vi "CRYSet Recall Front Panel.vi"(11 "Vi Ref":refnum<vi>) -> ()   [LabVIEW 2013]
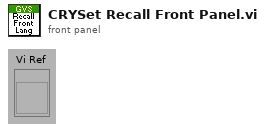
[diagram p1: front panel]
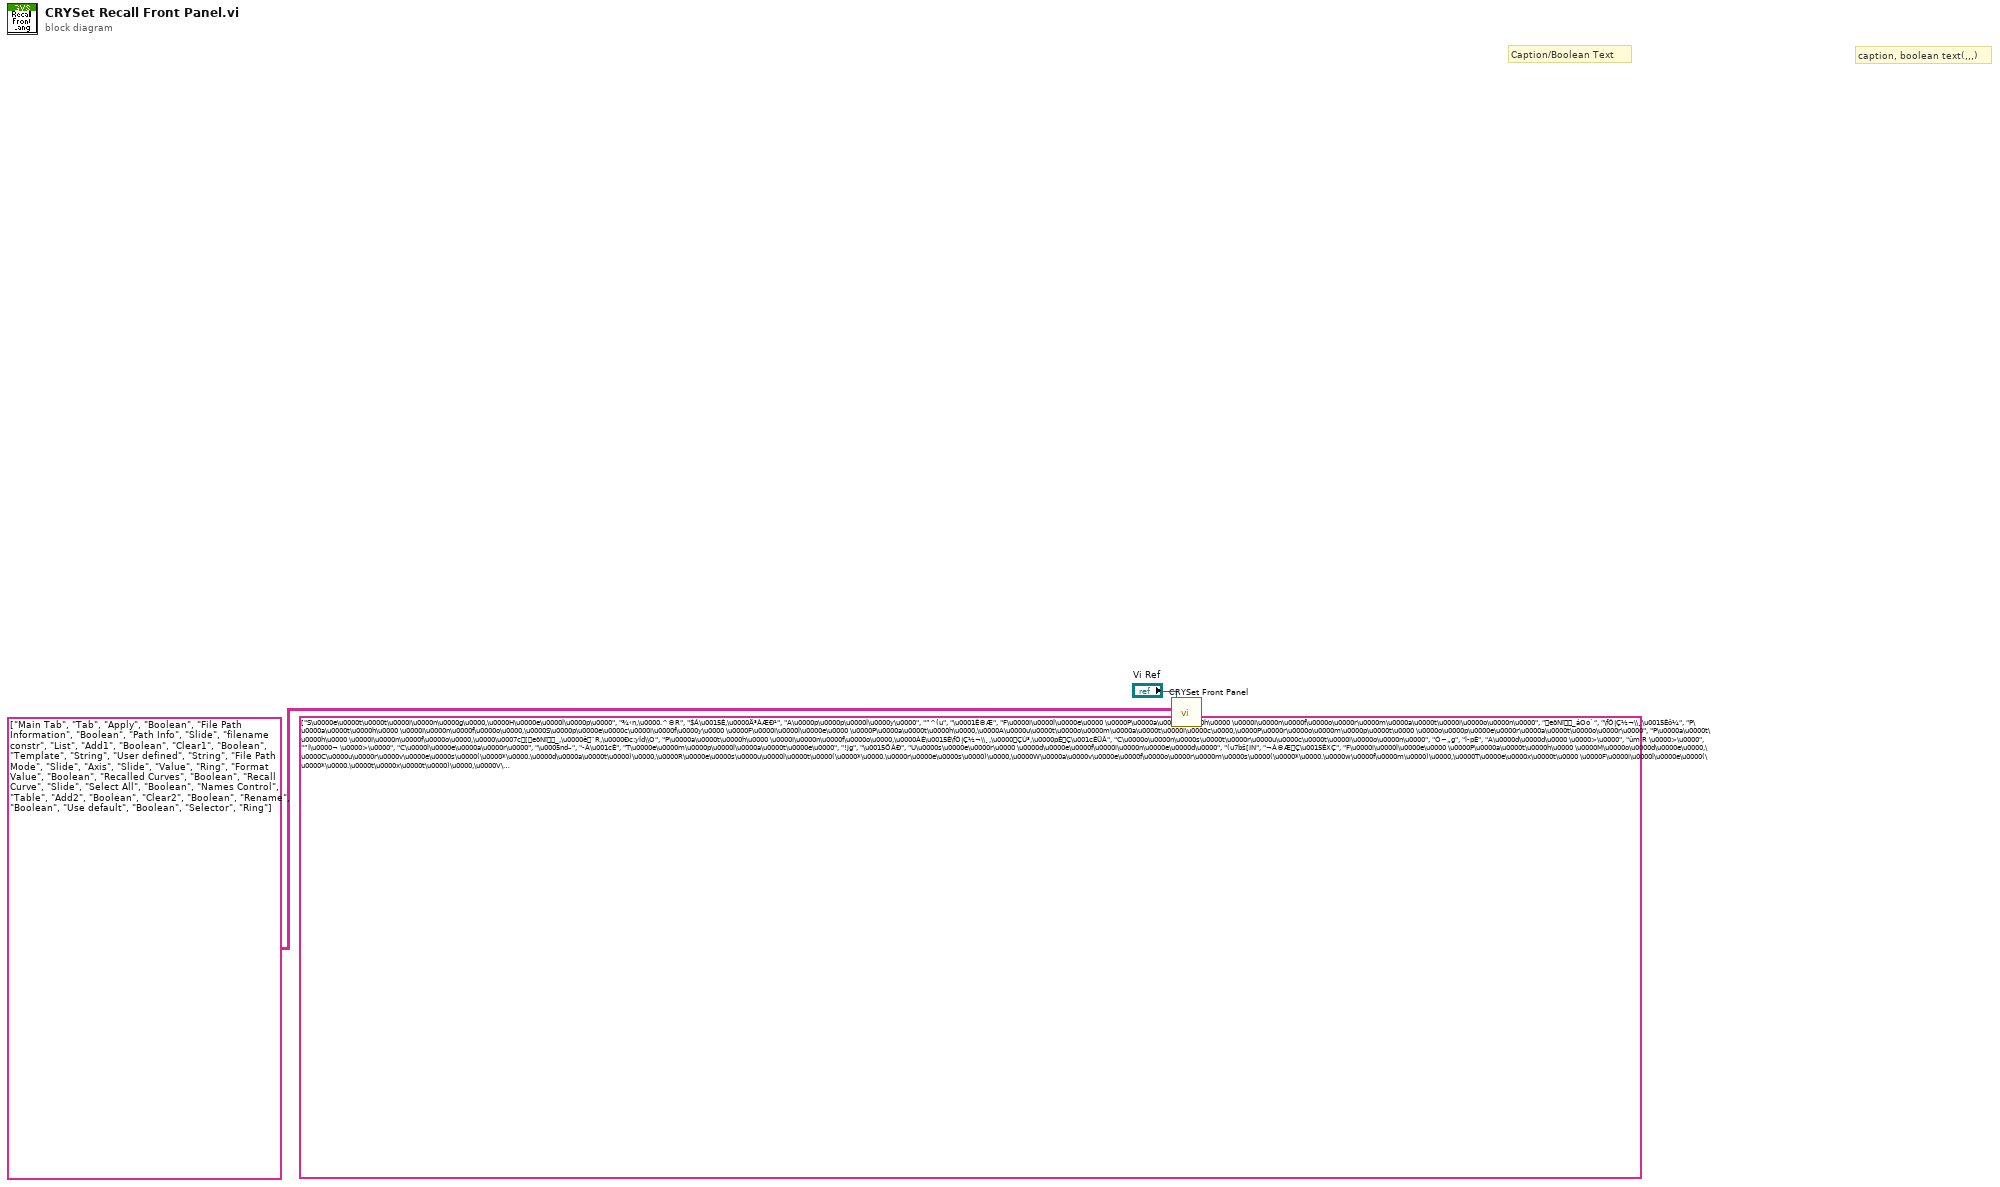
[diagram p0: block diagram]
diagram:
  # "Caption, Tab Page, Multilist Header, Button 4"
  # "Control Type"
  # "Control Name and Tab"
  # "caption, boolean text(,,,)"
  # "Caption/Boolean Text"
  n1 = call "CRYSet Front Panel.vi"("Caption(Boolean Text)"=string[][] [["S\u0000e\u0000t\u0000t\u0000i\u0000n\u0000g\u0000,\u0000H\u0000e\u0000l\u0000p\u0000", "¾‹n,\u0000.^©R", "$Á\u0015È,\u0000Ä³ÀÆÐ¹"], ["A\u0000p\u0000p\u0000l\u0000y\u0000", "”^(u", "\u0001È©Æ"], ["F\u0000i\u0000l\u0000e\u0000 \u0000P\u0000a\u0000t\u0000h\u0000 \u0000I\u0000n\u0000f\u0000o\u0000r\u0000m\u0000a\u0000t\u0000i\u0000o\u0000n\u0000", "eöNï_áOo`", "\fÓ|Ç½¬\\¸\u0015Èô¼"], ["P\u0000a\u0000t\u0000h\u0000 \u0000I\u0000n\u0000f\u0000o\u0000,\u0000S\u0000p\u0000e\u0000c\u0000i\u0000f\u0000y\u0000 \u0000F\u0000i\u0000l\u0000e\u0000 \u0000P\u0000a\u0000t\u0000h\u0000,\u0000A\u0000u\u0000t\u0000o\u0000m\u0000a\u0000t\u0000i\u0000c\u0000,\u0000P\u0000r\u0000o\u0000m\u0000p\u0000t\u0000 \u0000o\u0000p\u0000e\u0000r\u0000a\u0000t\u0000o\u0000r\u0000", "P\u0000a\u0000t\u0000h\u0000 \u0000I\u0000n\u0000f\u0000o\u0000,\u0000\u0007c[eöNï_,\u0000ê¨R,\u0000Ðc:yÍd\\O", "P\u0000a\u0000t\u0000h\u0000 \u0000I\u0000n\u0000f\u0000o\u0000,\u0000ÀÉ\u0015È\fÓ|Ç½¬\\¸,\u0000ÇÙ³,\u0000pÈÇ\u001cÈÜÂ"], ["C\u0000o\u0000n\u0000s\u0000t\u0000r\u0000u\u0000c\u0000t\u0000i\u0000o\u0000n\u0000", "Ó~„g", "l­pÈ"], ["A\u0000d\u0000d\u0000 \u0000>\u0000", "ûm R \u0000>\u0000", "”Í\u0000¬ \u0000>\u0000"], ["C\u0000l\u0000e\u0000a\u0000r\u0000", "\u0005nd–", "­À\u001cÈ"], ["T\u0000e\u0000m\u0000p\u0000l\u0000a\u0000t\u0000e\u0000", "!jg", "\u0015ÖÀÐ"], ["U\u0000s\u0000e\u0000r\u0000 \u0000d\u0000e\u0000f\u0000i\u0000n\u0000e\u0000d\u0000", "(u7bš[IN", "¬À©ÆÇ\u0015ÈXÇ"], ["F\u0000i\u0000l\u0000e\u0000 \u0000P\u0000a\u0000t\u0000h\u0000 \u0000M\u0000o\u0000d\u0000e\u0000,\u0000C\u0000u\u0000r\u0000v\u0000e\u0000s\u0000(\u0000*\u0000.\u0000d\u0000a\u0000t\u0000)\u0000,\u0000R\u0000e\u0000s\u0000u\u0000l\u0000t\u0000(\u0000*\u0000.\u0000r\u0000e\u0000s\u0000)\u0000,\u0000W\u0000a\u0000v\u0000e\u0000f\u0000o\u0000r\u0000m\u0000s\u0000(\u0000*\u0000.\u0000w\u0000f\u0000m\u0000)\u0000,\u0000T\u0000e\u0000x\u0000t\u0000 \u0000F\u0000i\u0000l\u0000e\u0000(\u0000*\u0000.\u0000t\u0000x\u0000t\u0000)\u0000,\u0000V\u0000a\u0000l\u0000u\u0000e\u0000(\u0000*\u0000.\u0000d\u0000a\u0000t\u0000)\u0000", "F\u0000i\u0000l\u0000e\u0000 \u0000P\u0000a\u0000t\u0000h\u0000 \u0000M\u0000o\u0000d\u0000e\u0000,\u0000òf¿~(\u0000*\u0000.\u0000d\u0000a\u0000t\u0000)\u0000,\u0000Ó~œg(\u0000*\u0000.\u0000r\u0000e\u0000s\u0000)\u0000,\u0000âlb_(\u0000*\u0000.\u0000w\u0000f\u0000m\u0000)\u0000,\u0000‡e,g‡eöN(\u0000*\u0000.\u0000t\u0000x\u0000t\u0000)\u0000,\u0000US<P(\u0000*\u0000.\u0000d\u0000a\u0000t\u0000)\u0000", "F\u0000i\u0000l\u0000e\u0000 \u0000P\u0000a\u0000t\u0000h\u0000 \u0000M\u0000o\u0000d\u0000e\u0000,\u0000á¬ Á(\u0000*\u0000.\u0000d\u0000a\u0000t\u0000)\u0000,\u0000°¬ü¬(\u0000*\u0000.\u0000r\u0000e\u0000s\u0000)\u0000,\u0000ÜÂ\u0004¬\fÓ\u0015Ö(\u0000*\u0000.\u0000w\u0000f\u0000m\u0000)\u0000,\u0000ø¼8»\fÓ|Ç(\u0000*\u0000.\u0000t\u0000x\u0000t\u0000)\u0000,\u0000\u0010È(\u0000*\u0000.\u0000d\u0000a\u0000t\u0000)\u0000"], ["A\u0000x\u0000i\u0000s\u0000,\u0000x\u0000,\u0000y\u0000,\u0000z\u0000", "t,\u0000x\u0000,\u0000y\u0000,\u0000z\u0000", "•Í,\u0000x\u0000,\u0000y\u0000,\u0000z\u0000"], ["V\u0000a\u0000l\u0000u\u0000e\u0000", "<P", "\u0012¬"], ["F\u0000o\u0000r\u0000m\u0000a\u0000t\u0000 \u0000V\u0000a\u0000l\u0000u\u0000e\u0000", "<h\u000f_<P", "\u0012¬\bÍ0®TÖ"], ["R\u0000e\u0000c\u0000a\u0000l\u0000l\u0000e\u0000d\u0000 \u0000C\u0000u\u0000r\u0000v\u0000e\u0000s\u0000", "\u0003Œ(uòf¿~", "¬Ç8ÖœÍá¬ Á"], ["R\u0000e\u0000c\u0000a\u0000l\u0000l\u0000:\u0000,\u0000S\u0000e\u0000l\u0000e\u0000c\u0000t\u0000i\u0000o\u0000n\u0000,\u0000L\u0000a\u0000s\u0000t\u0000 \u0000O\u0000n\u0000l\u0000y\u0000", "\u0003(u:\u0000,\u0000\téb,\u0000ÅN\u0000g\u000eT", "¬Ç8ÖœÍ:\u0000,\u0000 ÁÝÐ,\u0000\\Í…È\\Õ\u001c¬"], ["D\u0000e\u0000s\u0000e\u0000l\u0000e\u0000c\u0000t\u0000 \u0000A\u0000l\u0000l\u0000,\u0000S\u0000e\u0000l\u0000e\u0000c\u0000t\u0000 \u0000A\u0000l\u0000l\u0000", "ÖSm@b\tg,\u0000\téb@b\tg", "\u0004È´ÌèÍŒÁ,\u0000\u0004È´Ì ÁÝÐ"], ["C\u0000u\u0000r\u0000v\u0000e\u0000 \u0000o\u0000r\u0000 \u0000R\u0000e\u0000s\u0000u\u0000l\u0000t\u0000 \u0000N\u0000a\u0000m\u0000e\u0000s\u0000 \u0000t\u0000o\u0000 \u0000b\u0000e\u0000 \u0000R\u0000e\u0000c\u0000a\u0000l\u0000l\u0000e\u0000d\u0000", "\u0003Œ(u„vòf¿~\u0016bÓ~œg\rTW[", "¬Ç8ÖœÍ\u001c´ \u0000á¬ Á \u0000\u0010¶”² \u0000°¬ü¬tÇ„¹"], ["A\u0000d\u0000d\u0000 \u0000>\u0000", "ûm R \u0000>\u0000", "”Í\u0000¬ \u0000>\u0000"], ["C\u0000l\u0000e\u0000a\u0000r\u0000", "\u0005nd–", "­À\u001cÈ"], ["R\u0000e\u0000n\u0000a\u0000m\u0000e\u0000", "͑}T\rT", "tÇ„¹À¼½¬"], ["U\u0000s\u0000e\u0000 \u0000d\u0000e\u0000f\u0000a\u0000u\u0000l\u0000t\u0000", "(u7bš[IN", "0®\u0015È\u0012¬¬¹©Æ"], ["S\u0000e\u0000l\u0000e\u0000c\u0000t\u0000o\u0000r\u0000,\u0000S\u0000p\u0000a\u0000c\u0000e\u0000,\u0000U\u0000n\u0000d\u0000e\u0000r\u0000s\u0000c\u0000o\u0000r\u0000e\u0000s\u0000,\u0000N\u0000o\u0000n\u0000e\u0000", "\téb,\u0000zz<h,\u0000\u000bN\u0012R¿~,\u0000àe", " ÁÝÐÇ,\u0000S\u0000p\u0000a\u0000c\u0000e\u0000,\u0000U\u0000n\u0000d\u0000e\u0000r\u0000s\u0000c\u0000o\u0000r\u0000e\u0000s\u0000,\u0000N\u0000o\u0000n\u0000e\u0000"]], "Control ID and Type(Label Name, Type)"=string[][] [["Main Tab", "Tab"], ["Apply", "Boolean"], ["File Path Information", "Boolean"], ["Path Info", "Slide"], ["filename constr", "List"], ["Add1", "Boolean"], ["Clear1", "Boolean"], ["Template", "String"], ["User defined", "String"], ["File Path Mode", "Slide"], ["Axis", "Slide"], ["Value", "Ring"], ["Format Value", "Boolean"], ["Recalled Curves", "Boolean"], ["Recall Curve", "Slide"], ["Select All", "Boolean"], ["Names Control", "Table"], ["Add2", "Boolean"], ["Clear2", "Boolean"], ["Rename", "Boolean"], ["Use default", "Boolean"], ["Selector", "Ring"]], "Vi Ref"="Vi Ref") -> ()  [unwired: 9 in]
